vi "Get Ref.vi"(8 "error in (no error)":errorcluster, 11 "BetterTreeHandle in":refnum<class "BetterTreeHandle.lvclass">) -> (0 "error out":errorcluster, 2 "Tree/LB/MCL ref":refnum<vi>, 3 "BetterTreeHandle out":refnum<class "BetterTreeHandle.lvclass">)   [LabVIEW 2020, in "BetterDragAndDrop.lvlib" / "BetterTreeHandle.lvclass"]
uses:
  BetterTreeHandle.lvclass
  BetterTreeHandle.lvclass/BetterTreeHandle.ctl
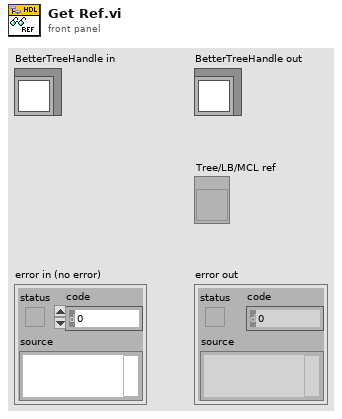
[diagram p1: front panel]
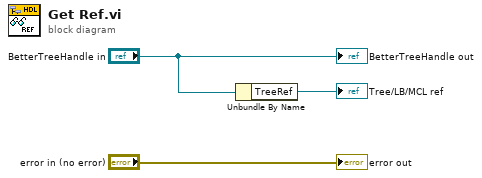
[diagram p0: block diagram]
diagram:
  n1 = Unbundle By Name("BetterTreeHandle in") -> ("TreeRef"=→"Tree/LB/MCL ref":refnum<vi>)
  "error out" <- "error in (no error)"
  "BetterTreeHandle out" <- "BetterTreeHandle in"
